vi "Angle Formatization.vi"(1 "Alpha":dbl) -> (0 "Alpha Formatized":dbl)   [LabVIEW 2012]
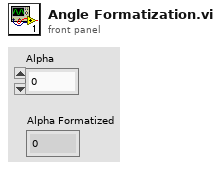
[diagram p1: front panel]
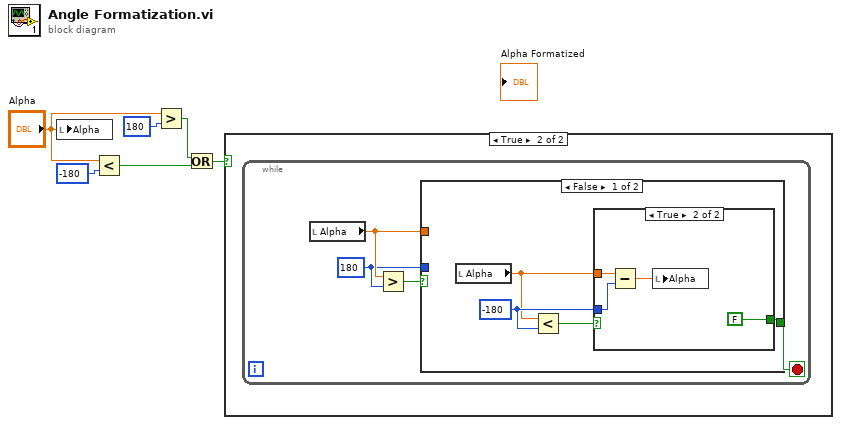
[diagram p0: block diagram]
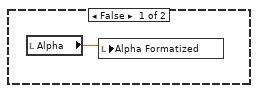
[diagram p2: hidden frame]
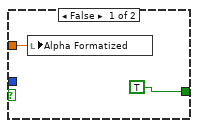
[diagram p3: hidden frame]
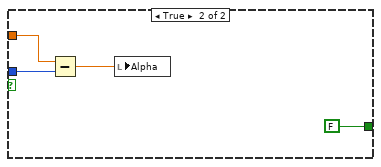
[diagram p4: hidden frame]
diagram:
  n1 = local write "Alpha"("Alpha") -> ()
  n2 = Less?(x="Alpha", y=-180) -> (x < y?=w3:bool)
  n3 = Greater?(x="Alpha", y=180) -> (0:w2:bool)
  n4 = Or(x=w2, y=w3) -> (x .or. y?=w1:bool)
  n5 = case shown="True" w1 {
    frame False {
      n6 = local read "Alpha"() -> (w7:dbl)
      n7 = local write "Alpha Formatized"(w7) -> ()
    }
    frame True {
      n8 = while {
        stop <- w8 stop-if-true
        w9 = 180
        n9 = local read "Alpha"() -> (w10:dbl)
        n10 = Greater?(x=w10, y=w9) -> (0:w11:bool)
        n11 = case shown="False" w11 {
          tunnel: w10 -> [_ w25]
          tunnel: w9 -> [_ w24]
          tunnel: [w12 FALSE] -> w8
          frame False {
            w14 = -180
            n12 = local read "Alpha"() -> (w13:dbl)
            n13 = Less?(x=w13, y=w14) -> (x < y?=w15:bool)
            n14 = case shown="True" w15 {
              tunnel: w14 -> [_ w21]
              tunnel: w13 -> [w17 w20]
              tunnel: [TRUE FALSE] -> w12
              frame False {
                n15 = local write "Alpha Formatized"(w17) -> ()
              }
              frame True {
                n16 = Subtract(x=w20, y=w21) -> (x-y=w19:dbl)
                n17 = local write "Alpha"(w19) -> ()
              }
            }
          }
          frame True {
            n18 = Subtract(x=w25, y=w24) -> (x-y=w23:dbl)
            n19 = local write "Alpha"(w23) -> ()
          }
        }
      }
    }
  }
